vi "UMLEditor_RemoveClassSuffix.vi"(11 "ObjectRuntimeClassName in":string) -> (3 "ObjectRuntimeClassName out":string)   [LabVIEW 2014]
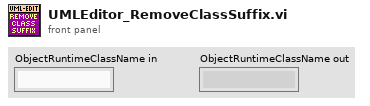
[diagram p1: front panel]
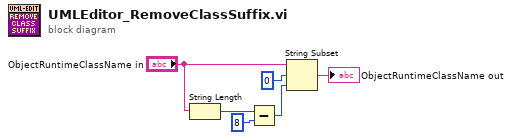
[diagram p0: block diagram]
diagram:
  n1 = String Length(string="ObjectRuntimeClassName in") -> (length=w2:i32)
  n2 = Subtract(x=w2, y=8) -> (x-y=w3:i32)
  n3 = String Subset(string="ObjectRuntimeClassName in", offset (0)=0, length (rest)=w3) -> (substring=→"ObjectRuntimeClassName out":string)
